vi "Build Video Arrays.vi"() -> (0 "Array High":u32[](array[numeric]), 1 "Array Medium":u32[](array[numeric]), 4 "Array Low":u32[](array[numeric]))   [LabVIEW 2015]
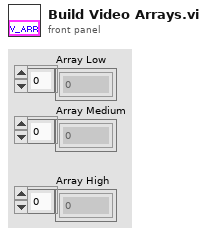
[diagram p1: front panel]
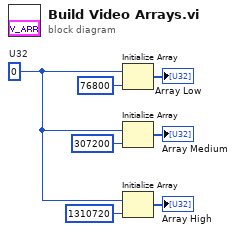
[diagram p0: block diagram]
diagram:
  w1 = u32 0  # U32
  n1 = Initialize Array(w1, 76800 ("dimension size")) -> (→"Array Low":u32[])
  n2 = Initialize Array(w1, 307200 ("dimension size")) -> (→"Array Medium":u32[])
  n3 = Initialize Array(w1, 1310720 ("dimension size")) -> (→"Array High":u32[])
